vi "libssh2_session_free.vi"(8 "error in (no error)":errorcluster, 11 "session":T1) -> (0 "error out":errorcluster, 3 "return value":i32)   [LabVIEW 2013, in "libssh2.lvlib"]
doc: "Frees all resources associated with a session instance."
uses:
  libssh2.lvlib
  Session Refnum.ctl
  libssh2.dll
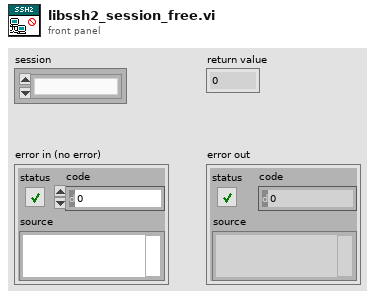
[diagram p1: front panel]
types:
  T1 = typedef "libssh2.lvlib/Session Refnum.ctl" = refnum<k1>
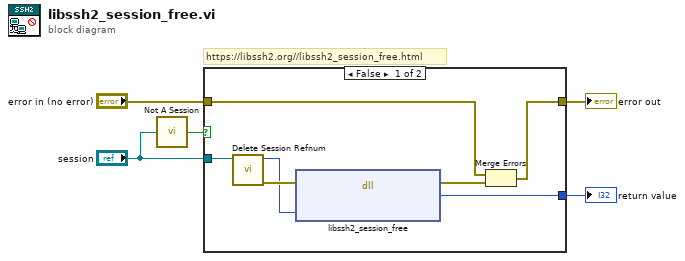
[diagram p0: block diagram]
diagram:
  # "https://libssh2.org//libssh2_session_free.html"
  n1 = call "Not A Session.vi"("session"="session") -> ("Not a Session?"=w1:bool)
  n2 = case shown="False" w1 {
    tunnel: [w12 _] -> w5
    tunnel: [w7 w13] -> w4
    tunnel: "error in (no error)" -> [w6 w13]
    tunnel: "session" -> [w8 _]
    frame False {
      n3 = call "Delete Session Refnum.vi"("Session"=w8) -> ("error out"=w10:errorcluster, "LIBSSH2_SESSION*"=w9:u64)  [unwired: 9 in]
      n4 = dll-call lib="C:/Users/pasca/source/repos/libssh2-labview/libssh2**.*" fn="libssh2_session_free"(error in=w10, "session"=w9) -> (error out=w11:errorcluster, "return value"=w12:i32)  [unwired: 3 in, 1 out]
      n5 = Merge Errors(w6, w11) -> (w7:errorcluster)
    }
    frame True {
    }
  }
  "return value" <- w5
  "error out" <- w4
